vi "LEDFlash.vi"(11 "Boolean":bool) -> ()   [LabVIEW 2013]
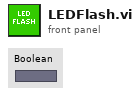
[diagram p1: front panel]
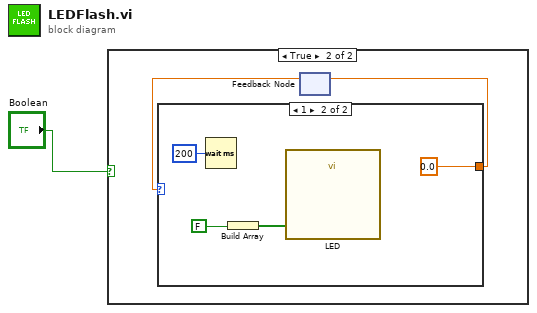
[diagram p0: block diagram]
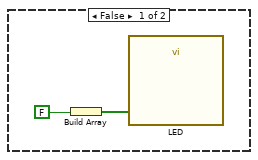
[diagram p2: hidden frame]
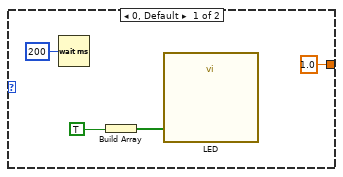
[diagram p3: hidden frame]
diagram:
  n1 = case shown="True" "Boolean" {
    frame False {
      n2 = Build Array(FALSE) -> (w2:bool[])
      n3 = call "LED"("data"=w2) -> ()  [unwired: 17 in, 2 out]
    }
    frame True {
      n4 = feedback #1() -> (w4:dbl)  [unwired: 1 in]
      n5 = case shown="1" w4 {
        tunnel: [1.0 0.0] -> w5
        frame 0, Default {
          n6 = Wait (ms)(milliseconds to wait=u32 200) -> ()  [unwired: 1 out]
          n7 = Build Array(TRUE) -> (w8:bool[])
          n8 = call "LED"("data"=w8) -> ()  [unwired: 17 in, 2 out]
        }
        frame 1 {
          n9 = Wait (ms)(milliseconds to wait=u32 200) -> ()  [unwired: 1 out]
          n10 = Build Array(FALSE) -> (w10:bool[])
          n11 = call "LED"("data"=w10) -> ()  [unwired: 17 in, 2 out]
        }
      }
      n12 = feedback-in #1(w5) -> ()
    }
  }
